vi "AlliGator Update Settings SEPL Parameters.vi"(6 "Gate Duration":dbl[unit], 8 "Error In":errorcluster, 9 "Gate Separation":dbl[unit], 10 "# Gates":u32, 11 "Gate Parameters Refnum":refnum<vi>) -> (0 "Error Out":errorcluster)   [LabVIEW 2021, in "AlliGator Settings.lvlib"]
doc: "Updates SEPL parameters in the Settings window."
uses:
  AlliGator Settings.lvlib
  Phasor/Phasor Explorer Gate Parameters.ctl
  Phasor/Phasor Gate Type.ctl
  Phasor/Phasor Type of User-defined Function.ctl
  Phasor/Phasor Explorer.lvlib
  Phasor/Phasor.lvlib
panel:
  # "see the AlliGator License on the block diagram (Ctrl+E or Window:Show Block Diagram)"
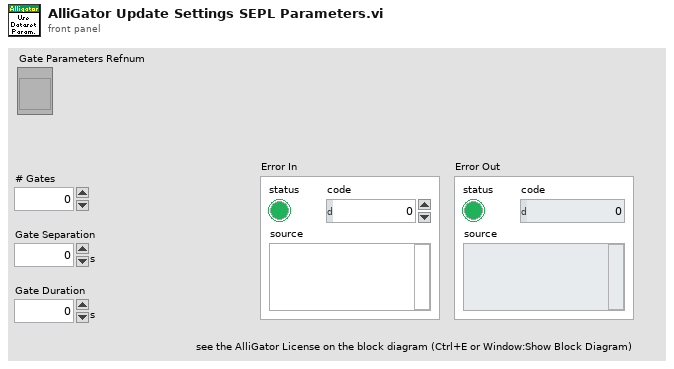
[diagram p1: front panel]
types:
  T1 = typedef "Phasor Explorer Gate Parameters.ctl" = cluster{"First Gate Start":dbl[unit], "Use Gate Center":bool, "Gate Width":dbl[unit], "Gate Step":dbl[unit], "# Gates":dbl, "Gate Type":T2, "Edge Width":dbl[unit], "Top Slope":dbl[unit], "Reversed Sawtooth?":bool, "Analytical Computation":bool, "Integration":enum32{"Item 0", "Item 1"}, "Tolerance":dbl, "# Steps":dbl, "Type of User-defined Function":T3, "Use Gate Step":bool}
  T2 = typedef "Gate Type.ctl" = enum16{"Square", "Finite Edge Square", "Finite Edge, Tilted Top Square", "Triangle", "Sawtooth", "User-defined"}
  T3 = typedef "Type of User-defined Function.ctl" = enum16{"Gate", "IRF"}
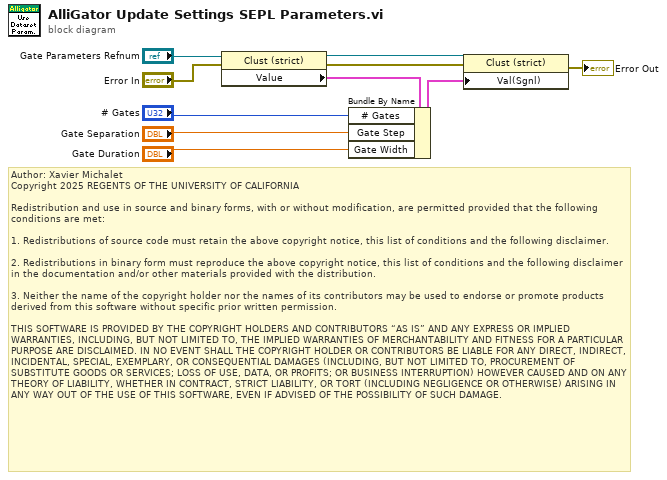
[diagram p0: block diagram]
diagram:
  # "Author: Xavier Michalet\nCopyright 2025 REGENTS OF THE UNIVERSITY OF CALIFORNIA\n\nRedistribution and use in source and binary forms, with or without modification, are permitted provided that the following conditions are met:\n\n1. Redistributions of source code must retain the above copyright notice, this list of conditions and the following disclaimer.\n\n2. Redistributions in binary form must reproduce the above copyright notice, this list of conditions and the following disclaimer in the documentation and/or other materials provided with the distribution.\n\n3. Neither the name of the copyright holder nor the names of its contributors may be used to endorse or promote products derived from this software without specific prior written permission.\n\nTHIS SOFTWARE IS PROVIDED BY THE COPYRIGHT HOLDERS AND CONTRIBUTORS “AS IS” AND ANY EXPRESS OR IMPLIED WARRANTIES, INCLUDING, BUT NOT LIMITED TO, THE IMPLIED WARRANTIES OF MERCHANTABILITY AND FITNESS FOR A PARTICULAR PURPOSE ARE DISCLAIMED. IN NO EVENT SHALL THE COPYRIGHT HOLDER OR CONTRIBUTORS BE LIABLE FOR ANY DIRECT, INDIRECT, INCIDENTAL, SPECIAL, EXEMPLARY, OR CONSEQUENTIAL DAMAGES (INCLUDING, BUT NOT LIMITED TO, PROCUREMENT OF SUBSTITUTE GOODS OR SERVICES; LOSS OF USE, DATA, OR PROFITS; OR BUSINESS INTERRUPTION) HOWEVER CAUSED AND ON ANY THEORY OF LIABILITY, WHETHER IN CONTRACT, STRICT LIABILITY, OR TORT (INCLUDING NEGLIGENCE OR OTHERWISE) ARISING IN ANY WAY OUT OF THE USE OF THIS SOFTWARE, EVEN IF ADVISED OF THE POSSIBILITY OF SUCH DAMAGE."
  n1 = property class="Clust (strict)"(reference="Gate Parameters Refnum", error in="Error In") -> (reference out=w4:refnum<vi>, error out=w3:errorcluster, "Value"=w8:T1)
  n2 = Bundle By Name(cluster=w8, "# Gates"="# Gates", "Gate Step"="Gate Separation", "Gate Width"="Gate Duration") -> (w2:T1)
  n3 = property class="Clust (strict)"(reference=w4, error in=w3, "Val(Sgnl)"=w2) -> (error out=→"Error Out":errorcluster)  [unwired: 1 out]
